vi "ReadWrite.Create.vi"(7 "Name":string, 8 "error in (no error)":errorcluster, 9 "Channel Refs":T1[](array[typedef]) format="%.0x", 10 "Custom Device Ref":T1 format="%.0x", 11 "Data Access API in":refnum<class "Data Access API.lvclass">) -> (0 "error out":errorcluster, 2 "Custom Device Ref out":T1 format="%.0x", 3 "Data Access API out":refnum<class "Data Access API.lvclass">)   [LabVIEW 2015, in "Data Access API.lvlib" / "Data Access API.lvclass"]
uses:
  Data Access API.lvclass
  <vilib>/NI Veristand/Custom Device API/Custom Device Item Ref.ctl
  Data/ReadWrite/ReadWrite.lvclass
  Data Access API.lvclass/Data Access API.ctl
  <vilib>/NI Veristand/Custom Device API/Custom Device API.lvlib
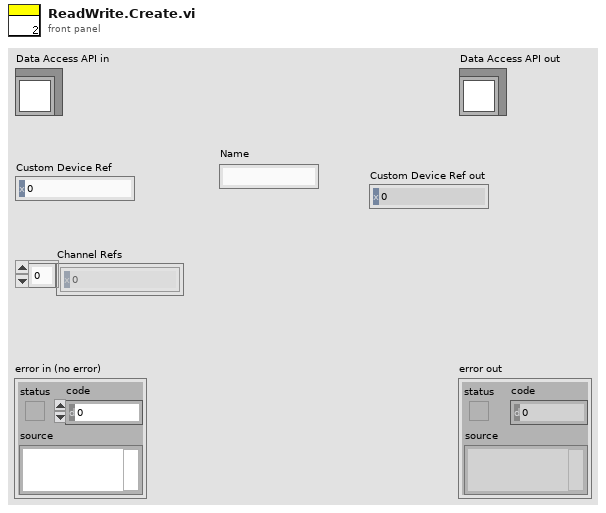
[diagram p1: front panel]
types:
  T1 = typedef "Custom Device API.lvlib/Custom Device Item Ref.ctl" = u64
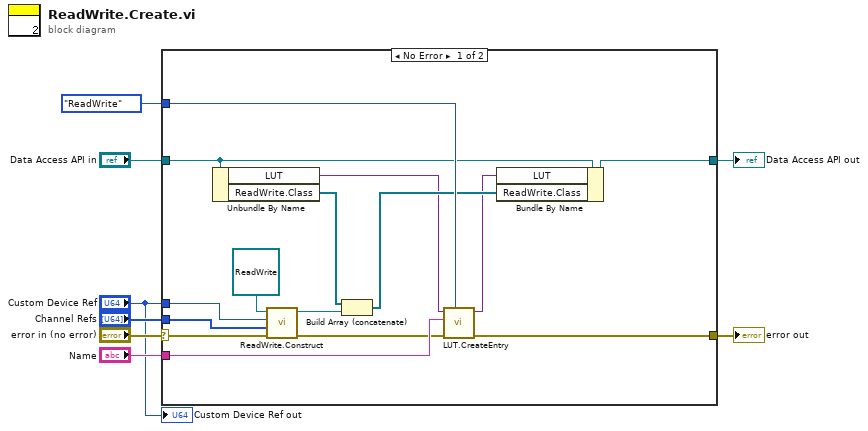
[diagram p0: block diagram]
diagram:
  n1 = case shown="No Error" "error in (no error)" {
    selector: "error in (no error)" -> [w20 w25]
    tunnel: [w19 w25] -> w7
    tunnel: [w21 w24] -> w5
    tunnel: "Data Access API in" -> [w22 w24]
    tunnel: enum16{"Read", "Write", "ReadWrite"}."ReadWrite" ("Type") -> [w23 _]
    tunnel: "Channel Refs" -> [w18 _]
    tunnel: "Custom Device Ref" -> [w17 _]
    tunnel: "Name" -> [w16 _]
    frame No Error {
      n2 = Unbundle By Name(w22) -> ("LUT"=w9:variant, "ReadWrite.Class"=w15:refnum<class "ReadWrite.lvclass">[])
      n3 = call "ReadWrite.Construct.vi"("error in (no error)"=w20, "Refs"=w18, "Parent"=w17, "ReadWrite in"=refnum<class "ReadWrite.lvclass"> refnum ("ReadWrite.lvclass")) -> ("error out"=w10:errorcluster, "ReadWrite out"=w13:refnum<class "ReadWrite.lvclass">)  [unwired: 6 in]
      n4 = Build Array (concatenate)(w15, w13) -> (w12:refnum<class "ReadWrite.lvclass">[])
      n5 = call "LUT.CreateEntry.vi"("Type"=w23, "error in (no error)"=w10, "Name"=w16, "LUT"=w9) -> ("error out"=w19:errorcluster, "LUT"=w11:variant)  [unwired: 6 in]
      n6 = Bundle By Name(cluster=w22, "LUT"=w11, "ReadWrite.Class"=w12) -> (w21:refnum<class "Data Access API.lvclass">)
    }
    frame Error {
    }
  }
  "error out" <- w7
  "Data Access API out" <- w5
  "Custom Device Ref out" <- "Custom Device Ref"
